vi "Set_Tunnel_Speed.vi"(3 "Mode":T1, 5 "Tunnel Velocity m/s":dbl min=0.0 max=50.0 format="%.2f") -> (0 "Error String":string)   [LabVIEW 2015]
doc: "This is an example of using features of the VI Server as a client. It shows how you might browse from one or more applications that may be exporting data from one or more data stations. \n\nThe example shows how to query a server for its list of exported VIs, how to get references to the VIs, and how call them with the Call By Reference function."
uses:
  Sub VIs/ADAM Controls/Tunnel_speed_mode.ctl
  Anemometry/Anemometry Sub Vis/File/Setup_Filetype.ctl
  Sub VIs/ADAM Controls/Update_scan_value.ctl
  Anemometry/Anemometry Sub Vis/Controls/Global_mode.ctl
  Sub VIs/ADAM Controls/Ch_description_ADAM.ctl
  Sub VIs/ADAM Controls/Module_type_ADAM.ctl
  Sub VIs/ADAM Controls/Function_ADAM.ctl
  Sub VIs/ADAM Controls/Channel_State.ctl
  Sub VIs/ADAM Controls/Calib_type_ADAM.ctl
  Sub VIs/ADAM Controls/Address.ctl
  <vilib>/Analysis/baseanly.llb/Mean (DBL).vi
  Anemometry/Anemometry Sub Vis/Globals/Preference_global.vi
  Anemometry/Anemometry Sub Vis/Globals/Trav_pos_global.vi
  Anemometry/Anemometry Sub Vis/Globals/Constants_global.vi
  <vilib>/Analysis/NI_AALBase.lvlib
panel:
  in  "Set EnFlo Tun Speed":refnum<vi>
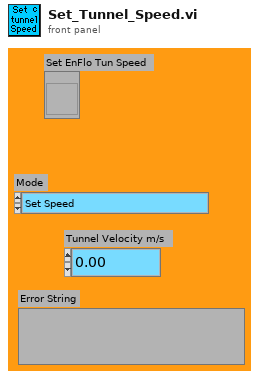
[diagram p1: front panel]
types:
  T1 = typedef "Tunnel_speed_mode.ctl" = enum16{"Set Speed", "Set Speed then wait", "Is tunnel speed allowable?"}
  T2 = typedef "Setup_Filetype.ctl" = enum16{"Measurement Setups", "Calibration Setups", "General", "Results File Plotter Setups", "Speed Calib Tweaks"}
  T3 = typedef "Channel_State.ctl" = enum16{"On", "Off", "Always On", "Always Off"}
  T4 = typedef "Calib_type_ADAM.ctl" = enum16{"Raw", "Bx + A", "Cx^2 + Bx + A", "Dx^3 + Cx^2 + Bx + A", "In Band", "Hi-Tec Q", "Hi-Tec M_dot", "Text"}
  T5 = typedef "Module_type_ADAM.ctl" = string
  T6 = typedef "Ch_description_ADAM.ctl" = cluster{"Ch Name":string, "Type":T5, "Function":T7, "Ch State":T3, "Calibration type":T4, "A":dbl, "B":dbl, "C":dbl, "D":dbl, "Comments":string, "Address":T8, "String":string, "Duty":u16}
  T7 = typedef "Function_ADAM.ctl" = enum16{"Analogue Input", "Digital Input", "Event counter", "Event rate", "Analogue Output", "Digital Output", "Relay Output"}
  T8 = typedef "Address.ctl" = cluster{"Main":i32, "Ch.":i32, "Sub":i32, "Port Name":string}
  T9 = typedef "Global_mode.ctl" = enum16{"Read Global", "Load Global From File", "Write Global to File"}
  T10 = typedef "Update_scan_value.ctl" = cluster{"Channel Name":string, "New Value":dbl}
  T11 = typedef "Server_Comms.ctl" = enum16{"Server Link Healthy", "Do Not Link To Server"}
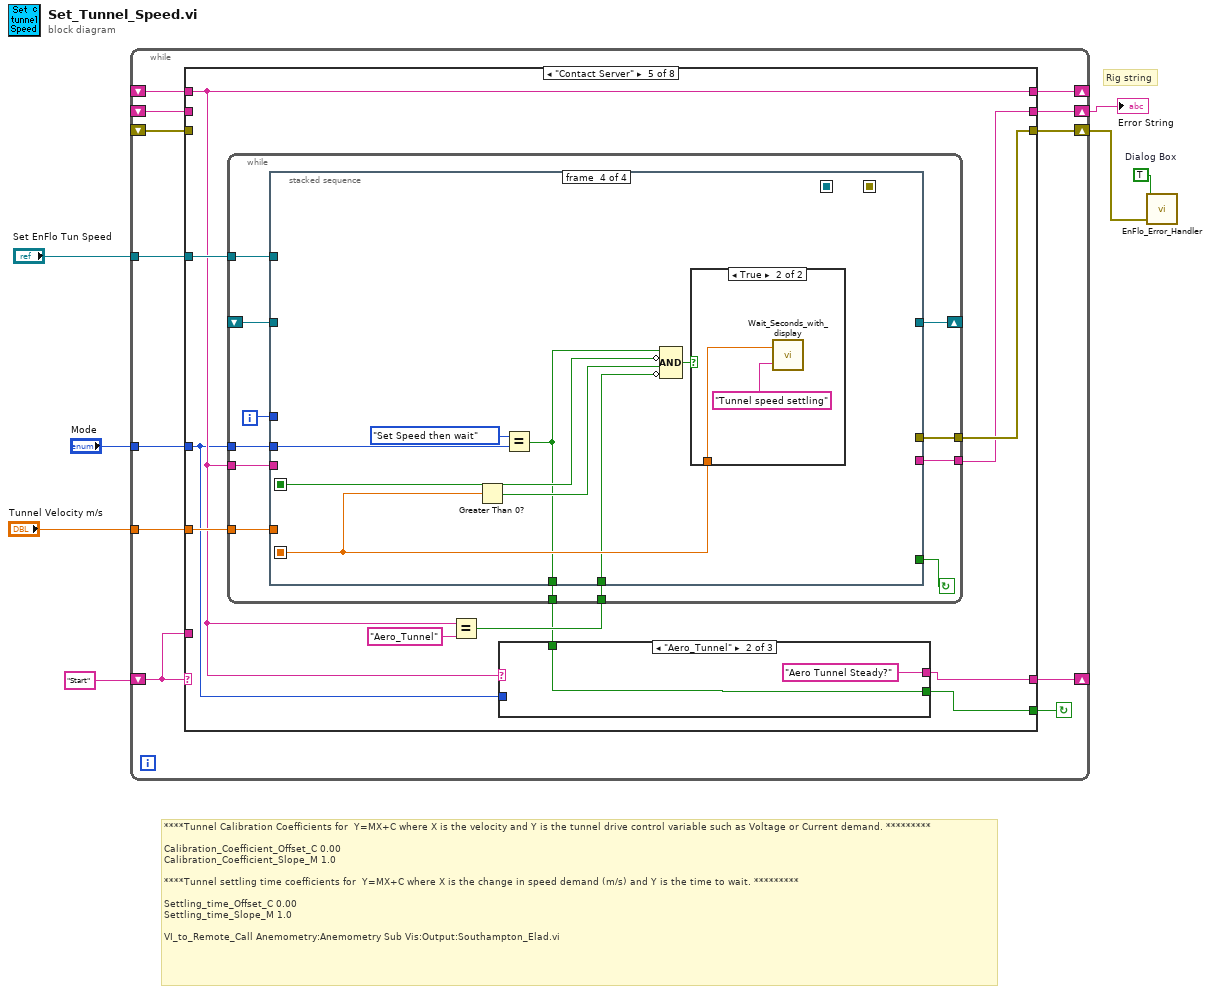
[diagram p0: block diagram]
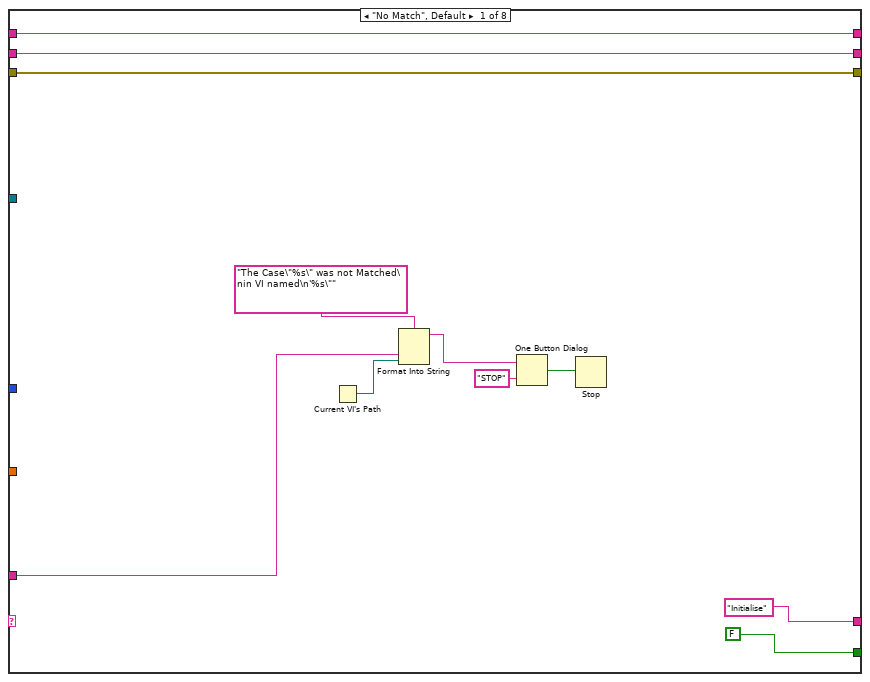
[diagram p2: hidden frame]
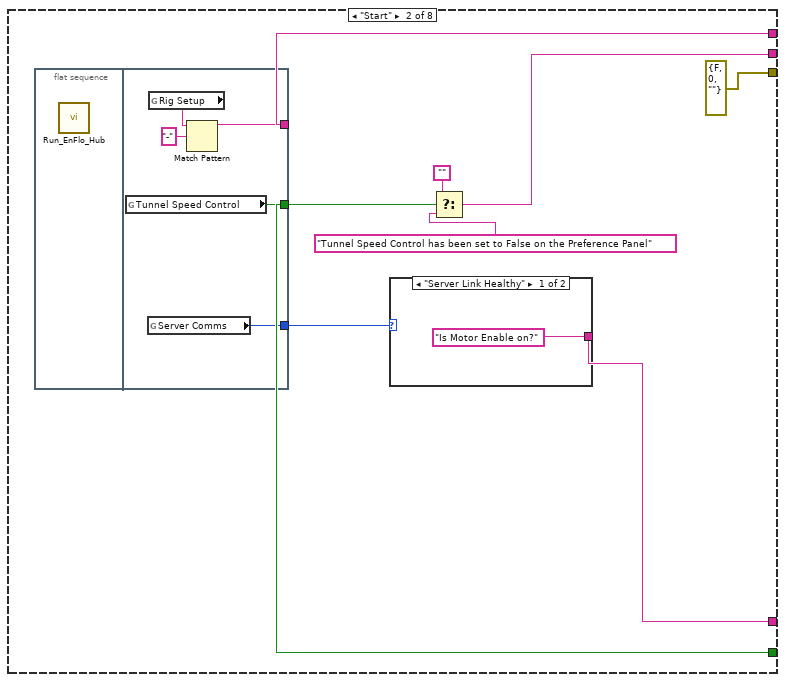
[diagram p3: hidden frame]
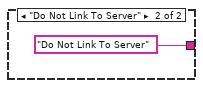
[diagram p4: hidden frame]
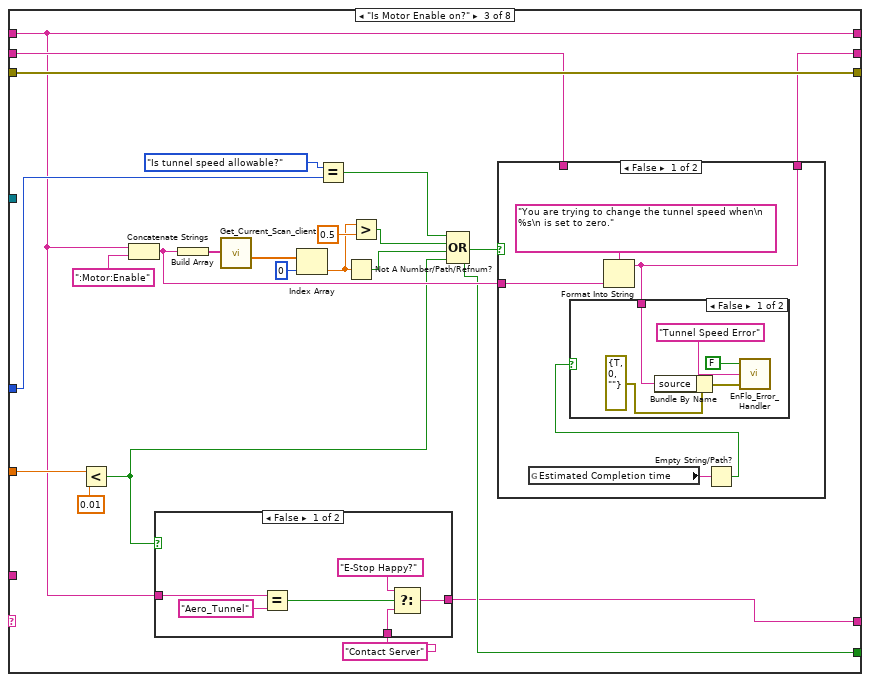
[diagram p5: hidden frame]
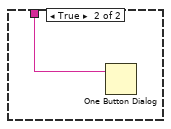
[diagram p7: hidden frame]
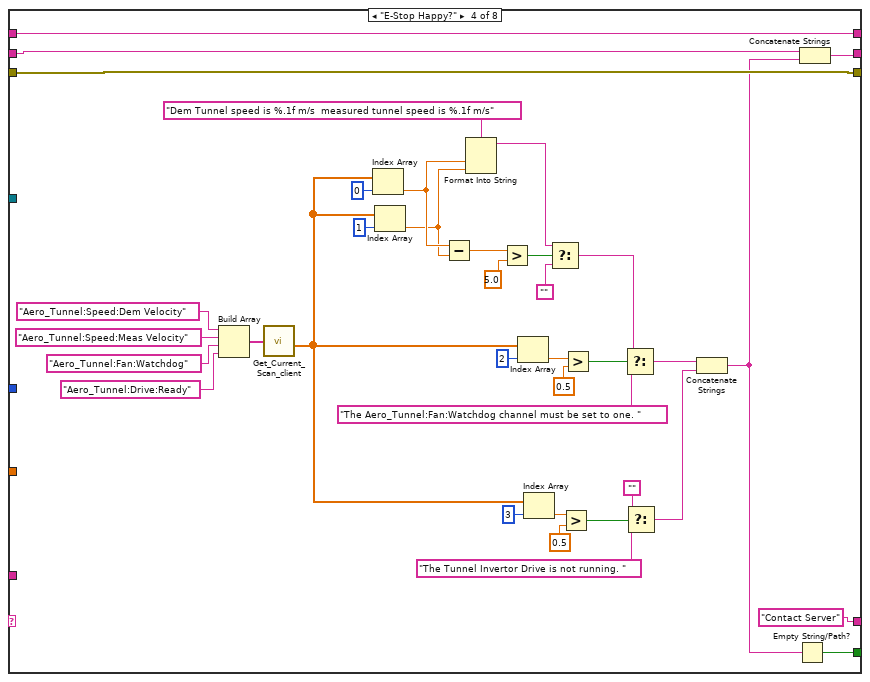
[diagram p9: hidden frame]
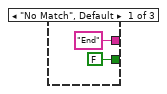
[diagram p10: hidden frame]
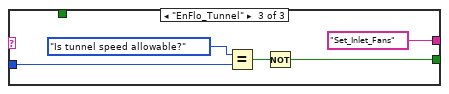
[diagram p11: hidden frame]
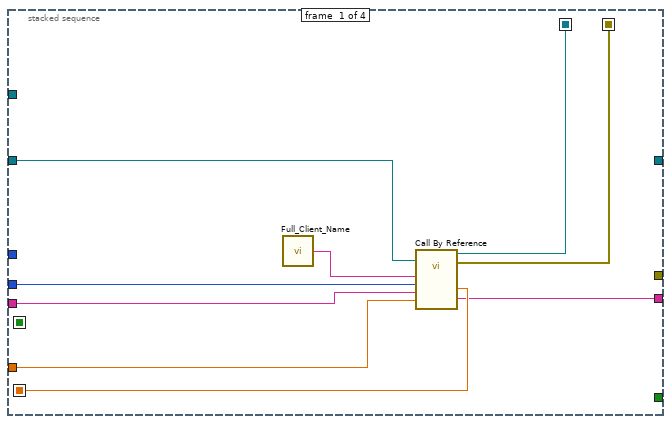
[diagram p12: hidden frame]
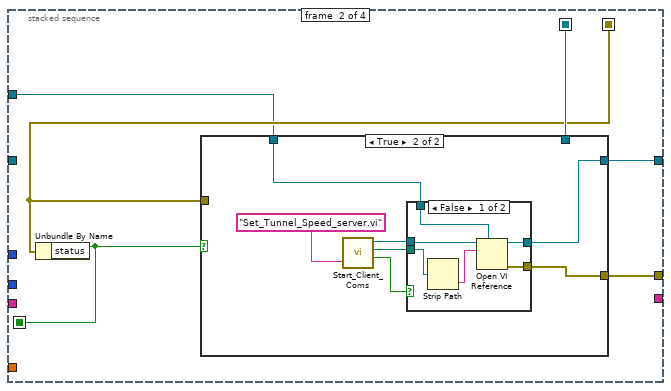
[diagram p13: hidden frame]
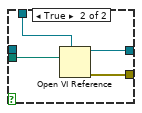
[diagram p15: hidden frame]
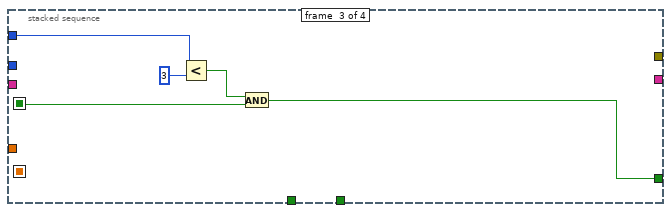
[diagram p16: hidden frame]
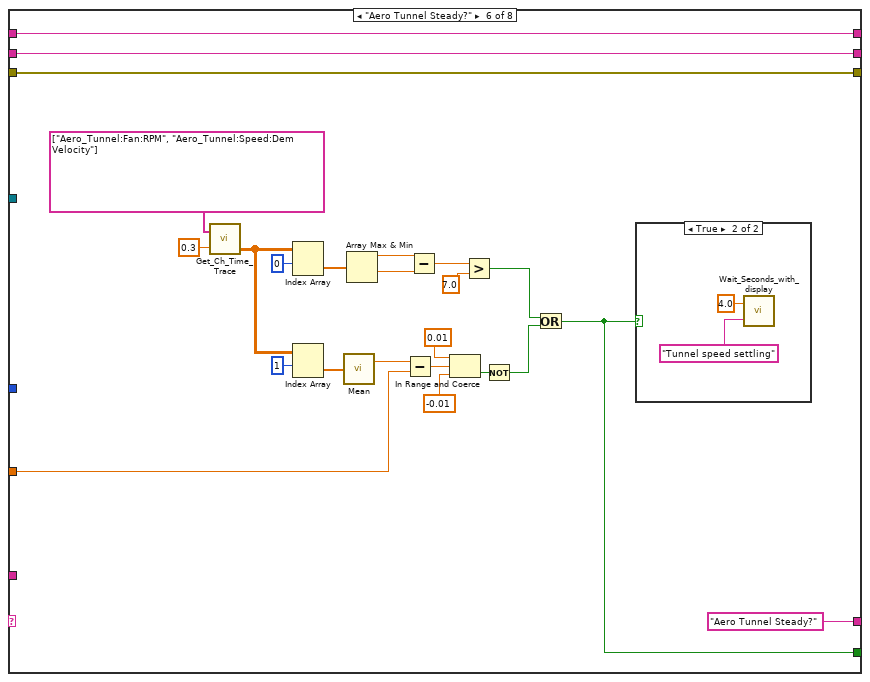
[diagram p18: hidden frame]
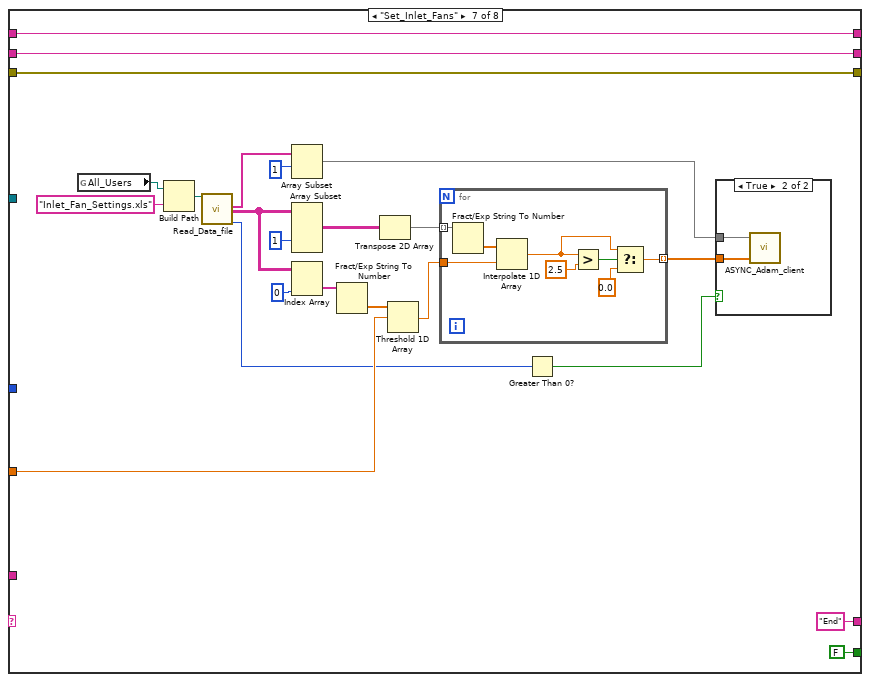
[diagram p20: hidden frame]
diagram:
  w7 = TRUE  # Dialog Box
  # "Rig string"
  # "****Tunnel Calibration Coefficients for  Y=MX+C where X is the velocity and Y is the tunnel drive control variable such as Voltage or Current demand. *********\n\nCalibration_Coefficient_Offset_C\t0.00\nCalibration_Coefficient_Slope_M\t1.0\n\n****Tunnel settling time coefficients for  Y=MX+C where X is the change in speed demand (m/s) and Y is the time to wait. *********\n\nSettling_time_Offset_C\t0.00\nSettling_time_Slope_M\t1.0\n\nVI_to_Remote_Call\tAnemometry:Anemometry Sub Vis:Output:Southampton_Elad.vi"
  n1 = while {
    shift-left: "Start" -> [w18]
    shift-right: [w19] -> _
    shift-right: [w17] -> w5
    shift-left: _ -> [w16]
    shift-right: [w15] -> w4
    shift-left: _ -> [w10]
    tunnel: "Mode" -> [w14]
    tunnel: "Tunnel Velocity m/s" -> [w13]
    shift-right: [w12] -> _
    shift-left: _ -> [w11]
    tunnel: "Set EnFlo Tun Speed" -> [w8]
    stop <- w9 continue-if-true
    n2 = case shown="\"Contact Server\"" w18 {
      tunnel: [FALSE w35 w53 w100 w126 w210 FALSE ("Tunnel Speed Control") FALSE] -> w9
      tunnel: ["Initialise" w31 w46 "Contact Server" ("f") w125 "Aero Tunnel Steady?" ("f") "End" ("f") "End"] -> w19
      tunnel: w18 -> [w25 _ _ _ _ _ _ _]
      tunnel: [w22 w33 w55 w114 w132 w226 w252 w266] -> w17
      tunnel: w16 -> [w22 _ w54 w115 _ w226 w252 _]
      tunnel: [w20 errorcluster {"status"=FALSE, "code"=0, "source"=""} ("error out") w57 w109 w133 w225 w251 w265] -> w15
      tunnel: w14 -> [_ _ w51 _ w124 _ _ w268]
      tunnel: w13 -> [_ _ w58 _ w134 w217 w233 w267]
      tunnel: [w21 w36 w49 w123 w127 w227 w253 w264] -> w12
      tunnel: w11 -> [w21 _ w49 w123 w127 w227 w253 w264]
      tunnel: w10 -> [w20 _ w57 w109 _ w225 w251 _]
      tunnel: w8 -> [_ _ _ _ w131 _ _ _]
      frame "No Match", Default {
        n3 = Current VI's Path() -> (path=w24:path)
        n4 = Format Into String(format string="The Case\"%s\" was not Matched\nin VI named\n'%s\"" ("Format String"), w25, w24) -> (resulting string=w28:string)  [unwired: 2 in, 1 out]
        n5 = One Button Dialog(message=w28, button name ("OK")="STOP") -> (true=w26:bool)
        n6 = Stop(stop? (T)=w26) -> ()
      }
      frame "Start" {
        n7 = flat-sequence {
          tunnel: [w45] -> w38
          tunnel: [w44] -> w35
          tunnel: [w41] -> w36
          frame #0 {
            n8 = call "Run_EnFlo_Hub.vi"() -> ()  [unwired: 8 out]
          }
          frame #1 {
            n9 = global read "Preference_global.vi" "Tunnel Speed Control"() -> (w44:bool)
            n10 = global read "Preference_global.vi" "Server Comms"() -> (w45:T11)
            n11 = global read "Preference_global.vi" "Rig Setup"() -> (w43:string)
            n12 = Match Pattern(string=w43, regular expression="-") -> (before substring=w41:string)  [unwired: 4 out]
          }
        }
        n13 = case shown="\"Server Link Healthy\"" w38 {
          tunnel: ["Is Motor Enable on?" "Do Not Link To Server"] -> w31
          frame "Server Link Healthy" {
          }
          frame "Do Not Link To Server" {
          }
        }
        n14 = Select(t="", s=w35, f="Tunnel Speed Control has been set to False on the Preference Panel" ("Error String")) -> (s? t:f=w33:string)
      }
      frame "Is Motor Enable on?" {
        n15 = Less?(x=w58, y=0.01) -> (x < y?=w48:bool)
        n16 = Concatenate Strings(w49, ":Motor:Enable" ("string")) -> (w56:string)
        n17 = case shown="False" w48 {
          tunnel: w49 -> [w72 _]
          tunnel: [w70 w74] -> w46
          tunnel: "Contact Server" ("f") -> [w68 w74]
          frame False {
            n18 = Equal?(x=w72, y="Aero_Tunnel") -> (x = y?=w71:bool)
            n19 = Select(t="E-Stop Happy?" ("f"), s=w71, f=w68) -> (s? t:f=w70:string)
          }
          frame True {
          }
        }
        n20 = Build Array(w56) -> (w60:string[])
        n21 = call "Get_Current_Scan_client.vi"("ADAM Ch Names"=w60) -> ("Numerical Values"=w61:dbl[])  [unwired: 3 out]
        n22 = Index Array(array=w61, index=0) -> (element=w63:dbl)
        n23 = Equal?(x=Tunnel_speed_mode."Is tunnel speed allowable?" ("Mode"), y=w51) -> (x = y?=w50:bool)
        n24 = Not A Number/Path/Refnum?(number/path/refnum=w63) -> (NaN/Path/Refnum?=w65:bool)
        n25 = Greater?(x=w63, y=0.5) -> (0:w66:bool)
        n26 = Compound Arithmetic op=OR(w50, w66, w65, w48) -> (w53:bool)
        n27 = case shown="False" w53 {
          tunnel: w56 -> [w78 _]
          tunnel: [w75 w86] -> w55
          tunnel: w54 -> [_ w86]
          frame False {
            n28 = global read "Trav_pos_global.vi" "Estimated Completion time"() -> (w77:string)
            n29 = Format Into String(format string="You are trying to change the tunnel speed when\n %s\n is set to zero.", w78) -> (resulting string=w75:string)  [unwired: 2 in, 1 out]
            n30 = Empty String/Path?(string/path=w77) -> (empty?=w76:bool)
            n31 = case shown="False" w76 {
              tunnel: w75 -> [w81 w85]
              frame False {
                n32 = Bundle By Name(cluster=errorcluster {"status"=TRUE, "code"=0, "source"=""} ("error in (no error)"), "source"=w81) -> (w82:errorcluster)
                n33 = call "EnFlo_Error_Handler.vi"("error in (no error)"=w82, "Error Type"="Tunnel Speed Error", "Dialog Box (T)"=FALSE) -> ()  [unwired: 3 out]
              }
              frame True {
                n34 = One Button Dialog(message=w85) -> ()  [unwired: 2 out]
              }
            }
          }
          frame True {
          }
        }
      }
      frame "E-Stop Happy?" {
        n35 = Build Array("Aero_Tunnel:Speed:Dem Velocity", "Aero_Tunnel:Speed:Meas Velocity", "Aero_Tunnel:Fan:Watchdog", "Aero_Tunnel:Drive:Ready") -> (w120:string[])
        n36 = call "Get_Current_Scan_client.vi"("ADAM Ch Names"=w120) -> ("Numerical Values"=w97:dbl[])  [unwired: 1 in, 2 out]
        n37 = Index Array(array=w97, index=0) -> (element=w113:dbl)
        n38 = Index Array(array=w97, index=1) -> (element=w112:dbl)
        n39 = Subtract(x=w113, y=w112) -> (x-y=w117:dbl)
        n40 = Format Into String(format string="Dem Tunnel speed is %.1f m/s  measured tunnel speed is %.1f m/s", w113, w112) -> (resulting string=w110:string)  [unwired: 2 in, 1 out]
        n41 = Greater?(x=w117, y=5.0) -> (0:w107:bool)
        n42 = Index Array(array=w97, index=2) -> (element=w104:dbl)
        n43 = Index Array(array=w97, index=3) -> (element=w96:dbl)
        n44 = Select(t=w110, s=w107, f="") -> (s? t:f=w102:string)
        n45 = Greater?(x=w96, y=0.5) -> (0:w94:bool)
        n46 = Greater?(x=w104, y=0.5) -> (0:w87:bool)
        n47 = Select(t=w102, s=w87, f="The Aero_Tunnel:Fan:Watchdog channel must be set to one. ") -> (s? t:f=w91:string)
        n48 = Select(t="", s=w94, f="The Tunnel Invertor Drive is not running. ") -> (s? t:f=w90:string)
        n49 = Concatenate Strings(w91, w90) -> (w89:string)
        n50 = Empty String/Path?(string/path=w89) -> (empty?=w100:bool)
        n51 = Concatenate Strings(w115, w89) -> (w114:string)
      }
      frame "Contact Server" {
        n52 = Equal?(x=w127, y="Aero_Tunnel") -> (x = y?=w129:bool)
        n53 = while {
          tunnel: w124 -> [w150]
          tunnel: w134 -> [w151]
          tunnel: [w152] -> w133
          shift-left: _ -> [w147]
          shift-right: [w155] -> _
          tunnel: [w149] -> w132
          tunnel: w127 -> [w148]
          tunnel: w131 -> [w146]
          tunnel: w129 -> [w145]
          tunnel: [w144] -> w128
          i -> [w154]
          stop <- w153 continue-if-true
          n54 = stacked-sequence {
            seq-local: [w163 _ _ _] -> [_ w169 _ _]
            seq-local: [w162 _ _ _] -> [_ w167 _ _]
            seq-local: [_ w168 _ _] -> [_ _ w191 w198]
            seq-local: [w159 _ _ _] -> [_ _ _ w201]
            tunnel: w147 -> [w164 _ _ _]
            tunnel: [_ w170 _ _] -> w155
            tunnel: w154 -> [_ _ w192 _]
            tunnel: [_ _ w190 _] -> w153
            tunnel: [_ w166 _ _] -> w152
            tunnel: w151 -> [w160 _ _ _]
            tunnel: w150 -> [w156 _ _ w202]
            tunnel: [w158 _ _ _] -> w149
            tunnel: w148 -> [w157 _ _ _]
            tunnel: w146 -> [_ w165 _ _]
            tunnel: w145 -> [_ _ _ w196]
            tunnel: [_ _ _ w195] -> w144
            frame #0 {
              n55 = call "Full_Client_Name.vi"() -> ("Client Name"=w161:string)
              n56 = call-by-ref "?"(reference=w164, "Tunnel Velocity m/s"=w160, "Rig Name"=w157, "Mode"=w156, "Client Name"=w161) -> (reference out=w163:refnum<vi>, error out=w162:errorcluster, "Error String"=w158:string, "Settling Time (s)"=w159:dbl)  [unwired: 1 in, 1 out]
            }
            frame #1 {
              n57 = Unbundle By Name(w167) -> ("status"=w168:bool)
              n58 = case shown="True" w168 {
                tunnel: [w171 w175] -> w170
                tunnel: w169 -> [w171 _]
                tunnel: [w172 w174] -> w166
                tunnel: w167 -> [w172 _]
                tunnel: w165 -> [_ w173]
                frame False {
                }
                frame True {
                  n59 = call "Start_Client_Coms.vi"("VI name to run on server"="Set_Tunnel_Speed_server.vi") -> ("LabVIEW application reference"=w177:refnum<vi>, "Checked VI name"=w178:path, "Local Call"=w176:bool)  [unwired: 1 in, 1 out]
                  n60 = case shown="False" w176 {
                    tunnel: [w184 w189] -> w175
                    tunnel: w173 -> [w182 w188]
                    tunnel: w178 -> [w181 w187]
                    tunnel: w177 -> [w180 _]
                    tunnel: [w183 w186] -> w174
                    frame False {
                      n61 = Strip Path(path=w181) -> (name=w185:string)  [unwired: 1 out]
                      n62 = Open VI Reference(type specifier VI Refnum (for type only)=w182, application reference (local)=w180, vi path=w185) -> (vi reference=w184:refnum<vi>, error out=w183:errorcluster)  [unwired: 1 in, 2 out]
                    }
                    frame True {
                      n63 = Open VI Reference(type specifier VI Refnum (for type only)=w188, vi path=w187) -> (vi reference=w189:refnum<vi>, error out=w186:errorcluster)  [unwired: 1 in, 3 out]
                    }
                  }
                }
              }
            }
            frame #2 {
              n64 = Less?(x=w192, y=3) -> (x < y?=w194:bool)
              n65 = And(x=w194, y=w191) -> (x .and. y?=w190:bool)
            }
            frame #3 {
              n66 = Greater Than 0?(x=w201) -> (x > 0?=w197:bool)
              n67 = Equal?(x=Tunnel_speed_mode."Set Speed then wait" ("Mode"), y=w202) -> (x = y?=w195:bool)
              n68 = Compound Arithmetic op=AND(w195, invert w198, w197, invert w196) -> (w199:bool)
              n69 = case shown="True" w199 {
                tunnel: w201 -> [_ w203]
                frame False {
                }
                frame True {
                  n70 = call "Wait_Seconds_with_display.vi"("Message"="Tunnel speed settling", "Seconds to wait"=w203) -> ()  [unwired: 2 out]
                }
              }
            }
          }
        }
        n71 = case shown="\"Aero_Tunnel\"" w127 {
          tunnel: w128 -> [_ w137 _]
          tunnel: [FALSE w137 w139] -> w126
          tunnel: ["End" ("f") "Aero Tunnel Steady?" ("f") "Set_Inlet_Fans" ("f")] -> w125
          tunnel: w124 -> [_ _ w141]
          frame "No Match", Default {
          }
          frame "Aero_Tunnel" {
          }
          frame "EnFlo_Tunnel" {
            n72 = Equal?(x=Tunnel_speed_mode."Is tunnel speed allowable?" ("Mode"), y=w141) -> (x = y?=w140:bool)
            n73 = Not(x=w140) -> (.not. x?=w139:bool)
          }
        }
      }
      frame "Aero Tunnel Steady?" {
        n74 = call "Get_Ch_Time_Trace.vi"("Desired Ch Names"=string[] ["Aero_Tunnel:Fan:RPM", "Aero_Tunnel:Speed:Dem Velocity"] ("ADAM Ch Names"), "History Length (mins)"=0.3) -> ("Output array"=w220:dbl[][])  [unwired: 2 out]
        n75 = Index Array(array=w220, index (row)=0) -> (element=w216:dbl[])  [unwired: 1 in]
        n76 = Index Array(array=w220, index (row)=1) -> (element=w219:dbl[])  [unwired: 1 in]
        n77 = call-poly <vilib>:"Mean.vi"("X"=w219) -> ("mean"=w218:dbl)  [unwired: 1 out]
        n78 = Array Max & Min(array=w216) -> (max value=w215:dbl, min value=w214:dbl)  [unwired: 2 out]
        n79 = Subtract(x=w218, y=w217) -> (x-y=w207:dbl)
        n80 = Subtract(x=w215, y=w214) -> (x-y=w213:dbl)
        n81 = In Range and Coerce(upper limit=0.01, x=w207, lower limit=-0.01) -> (In Range?=w206:bool)  [unwired: 1 out]
        n82 = Greater?(x=w213, y=7.0) -> (0:w211:bool)
        n83 = Not(x=w206) -> (.not. x?=w205:bool)
        n84 = Or(x=w211, y=w205) -> (x .or. y?=w210:bool)
        n85 = case shown="True" w210 {
          frame False {
          }
          frame True {
            n86 = call "Wait_Seconds_with_display.vi"("Message"="Tunnel speed settling", "Seconds to wait"=4.0) -> ()  [unwired: 2 out]
          }
        }
      }
      frame "Set_Inlet_Fans" {
        n87 = global read "Constants_global.vi" "All_Users"() -> (w238:path)
        n88 = Build Path(base path=w238, name or relative path="Inlet_Fan_Settings.xls") -> (appended path=w240:path)
        n89 = call "Read_Data_file.vi"("Results file"=w240) -> ("Ch names Out"=w246:string[], "Channel Values Out"=w242:string[][], "mark after read (chars.)"=w232:i32)  [unwired: 9 in, 7 out]
        n90 = Array Subset(array=w246, index=1) -> (w234:string[])  [unwired: 1 in]
        n91 = Array Subset(array=w242, index (col)=1 ("index")) -> (w237:string[][])  [unwired: 3 in]
        n92 = Index Array(array=w242, index (col)=0 ("index (row)")) -> (element=w244:string[])  [unwired: 1 in]
        n93 = Fract/Exp String To Number(string=w244) -> (number=w245:dbl[])  [unwired: 3 in, 1 out]
        n94 = Transpose 2D Array(2D array=w237) -> (transposed array=w236:string[][])
        n95 = Threshold 1D Array(2:w233, 3:w245) -> (0:w248:dbl)  [unwired: 1 in]
        n96 = for {
          tunnel: w236 -> [w263] mode=indexing
          tunnel: w248 -> [w262]
          tunnel: [w256] -> w235 mode=indexing
          n97 = Fract/Exp String To Number(string=w263) -> (number=w261:dbl[])  [unwired: 3 in, 1 out]
          n98 = Interpolate 1D Array(1:w262, 2:w261) -> (0:w258:dbl)
          n99 = Greater?(x=w258, y=2.5) -> (0:w259:bool)
          n100 = Select(t=w258, s=w259, f=0.0) -> (s? t:f=w256:dbl)
        }
        n101 = Greater Than 0?(x=w232) -> (x > 0?=w231:bool)
        n102 = case shown="True" w231 {
          tunnel: w235 -> [_ w255]
          tunnel: w234 -> [_ w254]
          frame False {
          }
          frame True {
            n103 = call "ASYNC_Adam_client.vi"("Values"=w255, "Channel Names"=w254) -> ()  [unwired: 1 in, 2 out]
          }
        }
      }
      frame "Do Not Link To Server" {
        # "Clamped"
        # "Pre vel"
        # "Tweak"
        # "Tweaked\nVel"
        # "Volts"
        n104 = stacked-sequence {
          seq-local: [w277 _ _ _ _ _ _] -> [_ w291 w297 w305 w321 w380 _]
          seq-local: [_ _ w292 _ _ _ _] -> [_ _ _ _ w325 _ _]
          seq-local: [_ _ _ w301 _ _ _] -> [_ _ _ _ w320 _ w393]
          seq-local: [_ _ _ w304 _ _ _] -> [_ _ _ _ w323 w375 _]
          seq-local: [_ _ _ _ w322 _ _] -> [_ _ _ _ _ w374 _]
          seq-local: [_ _ _ w306 _ _ _] -> [_ _ _ _ _ _ w399]
          seq-local: [w274 _ _ _ _ _ _] -> [_ _ _ _ _ _ w401]
          seq-local: [_ w282 _ _ _ _ _] -> [_ _ _ w299 _ _ w398]
          tunnel: w267 -> [_ w283 _ _ _ _ _]
          tunnel: w264 -> [w278 _ _ w314 _ _ w395]
          tunnel: w268 -> [_ _ _ _ w324 w369 _]
          tunnel: [_ w281 _ _ _ _ _] -> w266
          tunnel: [_ _ _ _ w319 _ _] -> w265
          frame #0 {
            n105 = Concatenate Strings(w278, "_Calib" ("Substring"), ".xls" ("string")) -> (w272:string)
            n106 = call "Setup_Filepath.vi"("Setup File Type"=Setup_Filetype."Speed Calib Tweaks", "Filename in"=w272) -> ("Filename Out"=w271:path)  [unwired: 1 out]
            n107 = call "Setup_Filepath.vi"("Setup File Type"=Setup_Filetype."Speed Calib Tweaks", "Filename in"="Current_Values.xls" ("name or relative path")) -> ("Filename Out"=w274:path)  [unwired: 1 out]
            n108 = call "Read_File_No_Error.vi"("Filename"=w271) -> ("string"=w277:string)  [unwired: 2 in, 7 out]
          }
          frame #1 {
            w285 = -2.0  # Min
            n109 = call "Get_value_from_string.vi"("Input string"=w291, "Variable name"="Maximum_Allowable_Tunnel_Speed") -> ("Value"=w284:dbl)  [unwired: 1 in, 1 out]
            n110 = In Range and Coerce(upper limit=w284, x=w283, lower limit=w285) -> (coerced(x)=w282:dbl)  [unwired: 1 out]
            n111 = Greater?(x=w283, y=w284) -> (0:w286:bool)
            n112 = Format Into String(format string="Req Speed Dem = %.1f m/s, Max allowable = %.1f m/s", w283, w284) -> (resulting string=w288:string)  [unwired: 2 in, 1 out]
            n113 = Select(t=w288, s=w286, f="") -> (s? t:f=w281:string)
          }
          frame #2 {
            n114 = call "Get_Characters_from_string.vi"("Input string"=w297, "Variable name"="VI_to_Remote_Call") -> ("Value"=w295:string)  [unwired: 1 in, 1 out]
            n115 = global read "Constants_global.vi" "EnFlo SW Folder"() -> (w293:path)
            n116 = call "String_to_Pathname.vi"("Input String"=w295) -> ("path"=w296:path)
            n117 = Path to Array of Strings(0:w296) -> (2:w294:string[])  [unwired: 1 out]
            n118 = call "Build_Pathname.vi"("PathElements"=w294, "PathnameIn"=w293) -> ("AppendedPath"=w292:path)
          }
          frame #3 {
            w312 = FALSE  # Tunnel Heated?
            n119 = local write "Tunnel Velocity m/s"(w299) -> ()
            n120 = call "Add_to_speed_calib_file.vi"("Desired Velocity"=w299, "Tunnel Heated?"=w312, "Rig Name"=w314, "Mode"=enum16{"Add Row", "Get Error Value"}."Get Error Value") -> ("Tweaked Demand"=w304:dbl, "Calib Tweak %"=w306:dbl)  [unwired: 2 in]
            n121 = Less?(x=w304, y=0.01) -> (x < y?=w302:bool)
            n122 = call "Get_value_from_string.vi"("Input string"=w305, "Variable name"="Calibration_Coefficient_Offset_C") -> ("Value"=w307:dbl)  [unwired: 1 in, 1 out]
            n123 = call "Get_value_from_string.vi"("Input string"=w305, "Variable name"="Calibration_Coefficient_Slope_M") -> ("Value"=w309:dbl)  [unwired: 1 in, 1 out]
            n124 = Multiply(x=w309, y=w304) -> (x*y=w308:dbl)
            n125 = Add(x=w307, y=w308) -> (x+y=w300:dbl)
            n126 = case shown="False" w302 {
              tunnel: w305 -> [_ w317]
              tunnel: [w315 w316] -> w301
              tunnel: w300 -> [w315 _]
              frame False {
              }
              frame True {
                n127 = call "Get_value_from_string.vi"("Input string"=w317, "Variable name"="Zero_Velocity_Output_Voltage") -> ("Value"=w316:dbl)  [unwired: 1 in, 1 out]
              }
            }
          }
          frame #4 {
            n128 = while {
              tunnel: w325 -> [w335]
              tunnel: w324 -> [w334]
              tunnel: w323 -> [w333]
              tunnel: [w332] -> w322
              shift-right: [w330] -> _
              shift-left: _ -> [w329]
              tunnel: [w328] -> w319
              tunnel: w321 -> [w327]
              tunnel: w320 -> [w326]
              stop <- TRUE stop-if-true
              n129 = case shown="\"Set Speed then wait\", Default" w334 {
                tunnel: w335 -> [_ w355]
                tunnel: w333 -> [_ w342]
                tunnel: [w337 w344] -> w332
                tunnel: [w337 w342] -> w330
                tunnel: w329 -> [w337 w343]
                tunnel: [errorcluster {"status"=FALSE, "code"=0, "source"=""} ("error out") w338] -> w328
                tunnel: w327 -> [_ _]
                tunnel: w326 -> [_ w341]
                frame "Is tunnel speed allowable?" {
                }
                frame "Set Speed then wait", Default {
                  n130 = Open VI Reference(type specifier VI Refnum (for type only)=refnum<vi> refnum, vi path=w355) -> (vi reference=w353:refnum<vi>, error out=w352:errorcluster)  [unwired: 1 in, 3 out]
                  n131 = property class="VI Interface Type 0"(reference=w353, error in=w352) -> (reference out=w350:refnum<vi>, error out=w351:errorcluster, "Front Panel.Open"=w349:bool)
                  n132 = case shown="False" w349 {
                    tunnel: w351 -> [w360 w363]
                    tunnel: w350 -> [w359 w364]
                    tunnel: [w358 w364] -> w348
                    tunnel: [w357 w363] -> w347
                    tunnel: [0.0 ("Tweaked Demand") w362] -> w344
                    tunnel: w343 -> [_ w362]
                    frame False {
                      n133 = property class="VI Interface Type 0"(reference=w359, error in=w360, "Front Panel.Open"=TRUE ("Front Panel Window:Open")) -> (reference out=w358:refnum<vi>, error out=w357:errorcluster)
                    }
                    frame True {
                    }
                  }
                  n134 = call-by-ref "?"(reference=w348, error in=w347, "Demand"=w341) -> (reference out=w345:refnum<vi>, error out=w346:errorcluster, "error out"=w339:errorcluster)
                  n135 = Close Reference(reference=w345, error in (no error)=w346) -> (error out=w340:errorcluster)
                  n136 = Select(t=w340, s=w340, f=w339) -> (s? t:f=w338:errorcluster)
                }
              }
            }
          }
          frame #5 {
            n137 = Subtract(x=w374, y=w375) -> (x-y=w373:dbl)
            n138 = Absolute Value(x=w373) -> (abs(x)=w367:dbl)
            n139 = call "Get_value_from_string.vi"("Input string"=w380, "Variable name"="Settling_time_Offset_C") -> ("Value"=w376:dbl)  [unwired: 1 in, 1 out]
            n140 = call "Get_value_from_string.vi"("Input string"=w380, "Variable name"="Settling_time_Slope_M") -> ("Value"=w378:dbl)  [unwired: 1 in, 1 out]
            n141 = Multiply(x=w378, y=w367) -> (x*y=w377:dbl)
            n142 = Add(x=w376, y=w377) -> (x+y=w368:dbl)
            n143 = Greater?(x=w367, y=0.05) -> (0:w365:bool)
            n144 = Equal?(x=Tunnel_speed_mode."Set Speed then wait" ("Mode"), y=w369) -> (x = y?=w371:bool)
            n145 = Compound Arithmetic op=AND(w365, w371) -> (w370:bool)
            n146 = case shown="False" w370 {
              tunnel: w368 -> [_ w382]
              frame False {
              }
              frame True {
                n147 = call "Wait_Seconds_with_display.vi"("Message"="Tunnel speed settling", "Seconds to wait"=w382) -> ()  [unwired: 2 out]
              }
            }
          }
          frame #6 {
            n148 = Concatenate Strings(w395, ":Speed:Dem_Voltage" ("string")) -> (w390:string)
            n149 = Bundle By Name(cluster=T6 {"Ch Name"="", "Type"="", "Function"=enum."Analogue Input", "Ch State"=enum."On", "Calibration type"=enum."Raw", "A"=0.0, "B"=0.0, "C"=0.0, "D"=0.0, "Comments"="", "Address"={"Main"=0, "Ch."=0, "Sub"=0, "Port Name"=""}, "String"="", "Duty"=0} ("Ch Discription"), "Ch Name"=w390, "Type"=T5 "Hold Value", "Calibration type"=Calib_type_ADAM."Raw", "Ch State"=Channel_State."On") -> (w384:T6)
            n150 = Bundle By Name(cluster=T10 {"Channel Name"="", "New Value"=0.0} ("Update Scan Value Cluster"), "Channel Name"=w390, "New Value"=w393) -> (w396:T10)
            n151 = call "Value_to_string.vi"("Value"=w399, "Label for value"="Calib Tweak") -> ("Output string"=w404:string)  [unwired: 1 in]
            n152 = call "Value_to_string.vi"("Value"=w398, "Label for value"="Velocity Demand") -> ("Output string"=w403:string)  [unwired: 1 in]
            n153 = Concatenate Strings(w404, w403) -> (w402:string)
            n154 = call "Write_File_Simple.vi"("append to file? (new file:F)"=FALSE, "character string"=w402, "file path"=w401) -> ()  [unwired: 2 out]
            n155 = Build Array(w384) -> (w385:T6[])
            n156 = Build Array(w396) -> (w386:T10[])
            n157 = call "Read_Write_Local_table.vi"("Mode"=Global_mode."Write Global to File", "Ch Values in"=w386, "Channels Descriptions In"=w385) -> ()  [unwired: 3 out]
          }
        }
      }
    }
  }
  "Error String" <- w5
  n158 = call "EnFlo_Error_Handler.vi"("error in (no error)"=w4, "Dialog Box (T)"=w7) -> ()  [unwired: 1 in, 3 out]
